vi "CV_test.vi"() -> ()   [LabVIEW 2015]
uses:
  Hardware libraries/Boonton7200/Boonton7200_IEEE-488_Bus_Mnemonics.ctl
  <vilib>/Analysis/1siggen.llb/Ramp Pattern by Delta.vi
  Hardware libraries/Boonton7200/Boonton7200.lvlib
  <vilib>/Analysis/NI_AALBase.lvlib
panel:
  in  "Zero":bool
  out "XY Graph 3":cluster{dbl[], dbl[]}(graph)
  out "XY Graph 2":cluster{dbl[], dbl[]}(graph)
  out "XY Graph":cluster{"Ramp Pattern":dbl[], dbl[]}(graph)
  out "1/C2-V":cluster{"Ramp Pattern":dbl[], dbl[]}(graph)
  out "Array":dbl[](array[numeric])
  in  "Hardware GPIB address":i32
  out "Error Out":errorcluster
  in  "Error In":errorcluster
  in  "Input parameters":T1
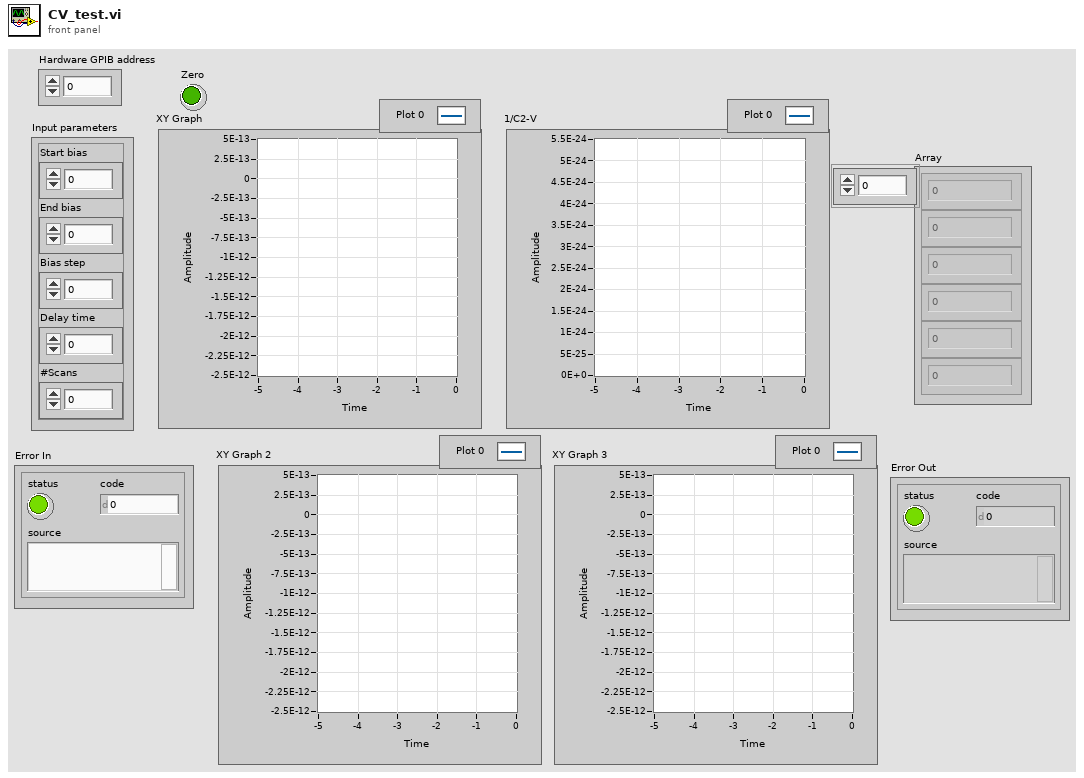
[diagram p1: front panel]
types:
  T1 = cluster{"Start bias":dbl, "End bias":dbl, "Bias step":dbl, "Delay time":u32, "#Scans":i32}
  T2 = typedef "Boonton7200_IEEE-488_Bus_Mnemonics.ctl" = string
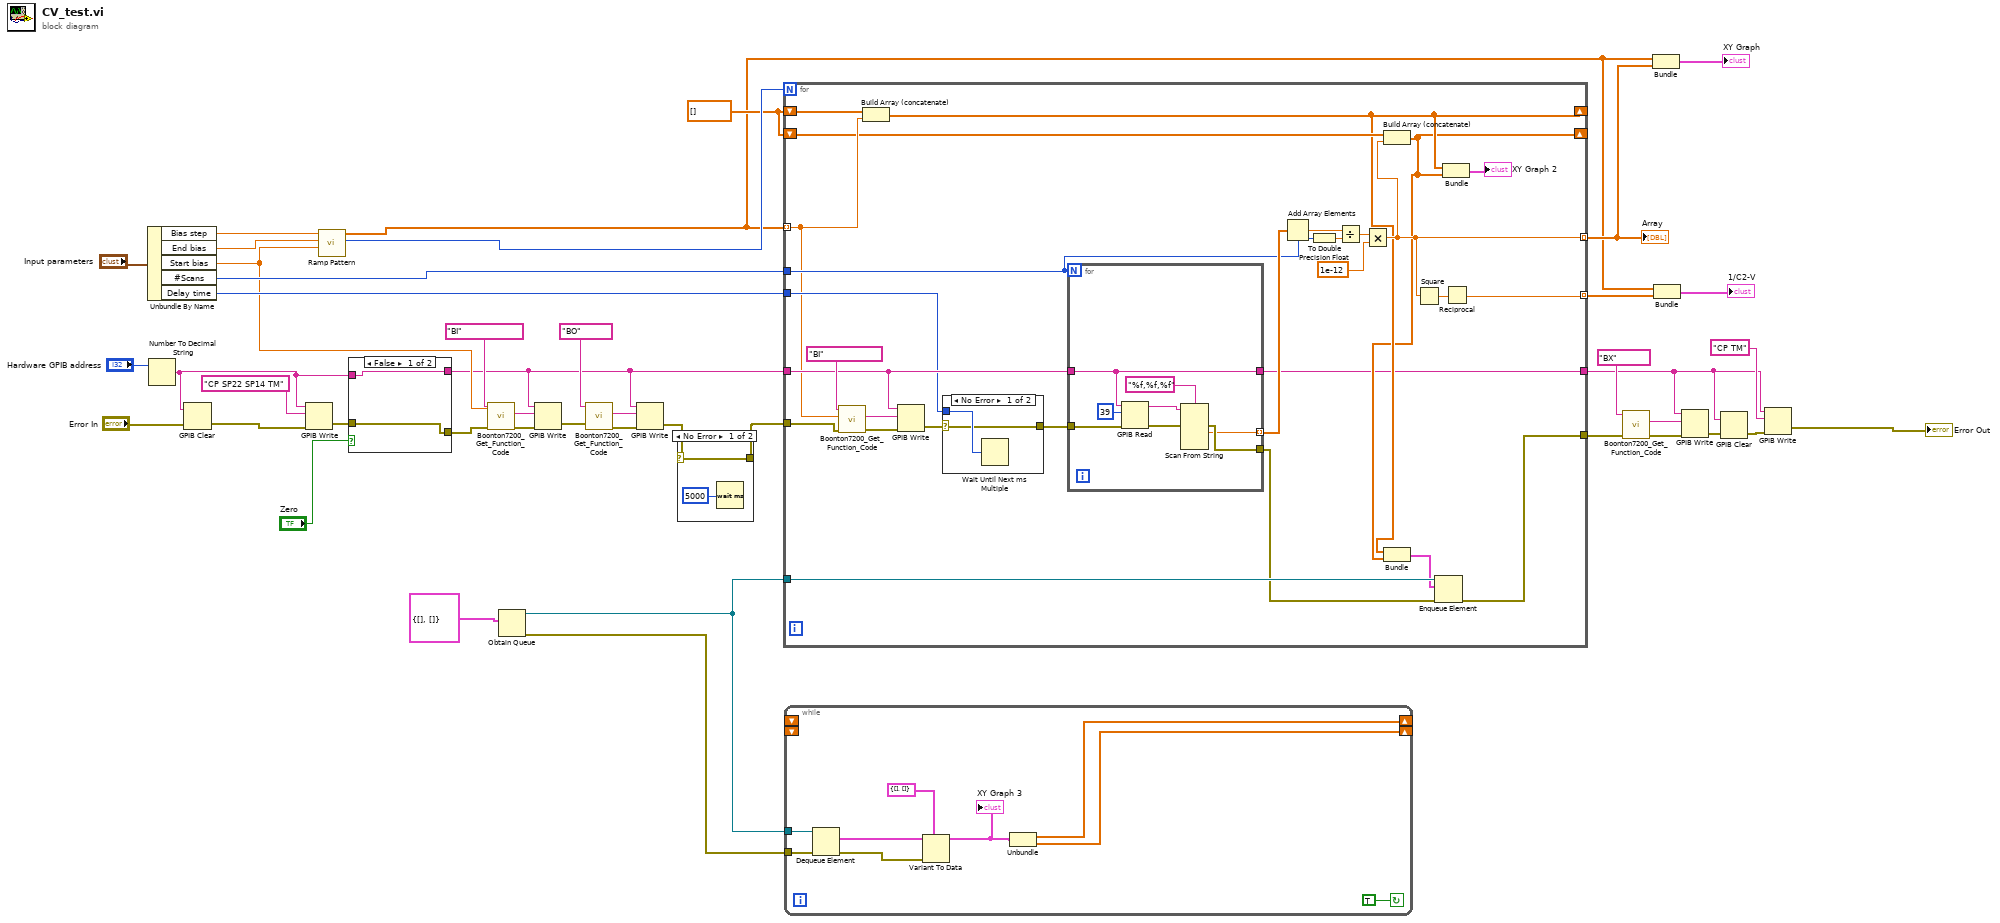
[diagram p0: block diagram]
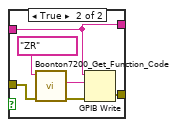
[diagram p2: hidden frame]
diagram:
  w15 = dbl[] []
  n1 = Unbundle By Name("Input parameters") -> ("Bias step"=w40:dbl, "End bias"=w39:dbl, "Start bias"=w31:dbl, "#Scans"=w37:i32, "Delay time"=w36:u32)
  n2 = Number To Decimal String(number="Hardware GPIB address") -> (decimal integer string=w3:string)  [unwired: 1 in]
  n3 = GPIB Clear(2:"Error In", 3:w3) -> (0:w34:errorcluster)  [unwired: 1 out]
  n4 = GPIB Write(0:w3, 1:"CP SP22 SP14 TM" ("data"), 3:w34) -> (6:w6:errorcluster)  [unwired: 2 in, 1 out]
  n5 = call-poly <vilib>:"Ramp Pattern.vi"("start"=w31, "end"=w39, "delta"=w40) -> ("samples"=w38:i32, "Ramp Pattern"=w12:dbl[])  [unwired: 6 in, 1 out]
  n6 = case shown="False" "Zero" {
    tunnel: w6 -> [w44 w50]
    tunnel: [w44 w48] -> w5
    tunnel: [w45 w47] -> w4
    tunnel: w3 -> [w45 w47]
    frame False {
    }
    frame True {
      n7 = call "Boonton7200_Get_Function_Code.vi"("Error In"=w50, "IEEE-488 Bus Mnemonics"=T2 "ZR") -> ("Error Out"=w49:errorcluster, "GPIB code (IEEE-488)"=w46:string)  [unwired: 8 in]
      n8 = GPIB Write(0:w47, 1:w46, 3:w49) -> (6:w48:errorcluster)  [unwired: 2 in, 1 out]
    }
  }
  n9 = call "Boonton7200_Get_Function_Code.vi"("Error In"=w5, "Data Value"=w31, "IEEE-488 Bus Mnemonics"=T2 "BI") -> ("Error Out"=w33:errorcluster, "GPIB code (IEEE-488)"=w23:string)  [unwired: 7 in]
  n10 = Obtain Queue(element data type=cluster{dbl[], dbl[]} {[], []}) -> (queue out=w14:refnum<queue>, error out=w13:errorcluster)  [unwired: 4 in, 1 out]
  n11 = GPIB Write(0:w4, 1:w23, 3:w33) -> (6:w30:errorcluster)  [unwired: 2 in, 1 out]
  n12 = call "Boonton7200_Get_Function_Code.vi"("Error In"=w30, "IEEE-488 Bus Mnemonics"=T2 "BO") -> ("Error Out"=w28:errorcluster, "GPIB code (IEEE-488)"=w22:string)  [unwired: 8 in]
  n13 = GPIB Write(0:w4, 1:w22, 3:w28) -> (6:w8:errorcluster)  [unwired: 2 in, 1 out]
  n14 = case shown="No Error" w8 {
    selector: w8 -> [w53 w54]
    tunnel: [w53 w54] -> w9
    frame No Error {
      n15 = Wait (ms)(milliseconds to wait=u32 5000) -> ()  [unwired: 1 out]
    }
    frame Error {
    }
  }
  n16 = for {
    N: w38 -> [_]
    tunnel: w12 -> [w65] mode=indexing
    tunnel: w37 -> [w75]
    tunnel: w36 -> [w71]
    tunnel: w4 -> [w79]
    tunnel: w9 -> [w78]
    tunnel: [w61] -> w27 mode=indexing
    tunnel: [w70] -> w24 mode=indexing
    shift-right: [w59] -> _
    shift-left: w15 -> [w66]
    shift-right: [w58] -> _
    shift-left: w15 -> [w64]
    tunnel: w14 -> [w62]
    tunnel: [w56] -> w10
    tunnel: [w55] -> w1
    n17 = call "Boonton7200_Get_Function_Code.vi"("Error In"=w78, "Data Value"=w65, "IEEE-488 Bus Mnemonics"=T2 "BI") -> ("Error Out"=w80:errorcluster, "GPIB code (IEEE-488)"=w74:string)  [unwired: 7 in]
    n18 = Build Array (concatenate)(w66, w65) -> (w59:dbl[])
    n19 = GPIB Write(0:w79, 1:w74, 3:w80) -> (6:w73:errorcluster)  [unwired: 2 in, 1 out]
    n20 = case shown="No Error" w73 {
      selector: w73 -> [w82 w84]
      tunnel: [w82 w84] -> w72
      tunnel: w71 -> [w83 _]
      frame No Error {
        n21 = Wait Until Next ms Multiple(millisecond multiple=w83) -> ()  [unwired: 1 out]
      }
      frame Error {
      }
    }
    n22 = for {
      N: w75 -> [_]
      tunnel: w72 -> [w92]
      tunnel: w79 -> [w85]
      tunnel: [w86] -> w77 mode=indexing
      tunnel: [w87] -> w60
      tunnel: [w85] -> w56
      n23 = GPIB Read(0:w85, 1:39 ("byte count"), 3:w92) -> (5:w90:string, 7:w88:errorcluster)  [unwired: 2 in, 1 out]
      n24 = Scan From String(format string="%f,%f,%f", input string=w90, error in=w88) -> (error out=w87:errorcluster, output 1=w86:dbl)  [unwired: 6 in, 2 out]
    }
    n25 = Add Array Elements(numeric array=w77) -> (sum=w76:dbl)
    n26 = To Double Precision Float(number=w75) -> (double precision float=w67:dbl)
    n27 = Divide(x=w76, y=w67) -> (x/y=w69:dbl)
    n28 = Multiply(x=w69, y=1e-12) -> (x*y=w61:dbl)
    n29 = Build Array (concatenate)(w64, w61) -> (w58:dbl[])
    n30 = Bundle(w59, w58) -> (w57:cluster{dbl[], dbl[]})  [unwired: 1 in]
    n31 = Square(x=w61) -> (x^2=w70:dbl)
    n32 = Enqueue Element(queue=w62, element=w57, error in (no error)=w60) -> (error out=w55:errorcluster)  [unwired: 1 in, 2 out]
    n33 = Bundle(w59, w58) -> (→"XY Graph 2":cluster{dbl[], dbl[]})  [unwired: 1 in]
    n34 = Reciprocal(x=w70) -> ()  [unwired: 1 out]
  }
  "Array" <- w27
  n35 = while {
    tunnel: w14 -> [w101]
    tunnel: w13 -> [w100]
    shift-right: [w95] -> _
    shift-left: _ -> [_]
    shift-right: [w94] -> _
    shift-left: _ -> [_]
    stop <- TRUE continue-if-true
    n36 = Dequeue Element(queue=w101, error in (no error)=w100) -> (element=w98:cluster{dbl[], dbl[]}, error out=w99:errorcluster)  [unwired: 1 in, 2 out]
    n37 = Variant To Data(error in=w99, type=cluster{dbl[], dbl[]} {[], []}, Variant=w98) -> (data=w96:cluster{dbl[], dbl[]})  [unwired: 1 out]
    "XY Graph 3" <- w96
    n38 = Unbundle(w96) -> (w94:dbl[], w95:dbl[])
  }
  n39 = call "Boonton7200_Get_Function_Code.vi"("Error In"=w1, "IEEE-488 Bus Mnemonics"=T2 "BX") -> ("Error Out"=w26:errorcluster, "GPIB code (IEEE-488)"=w21:string)  [unwired: 8 in]
  n40 = Bundle("Ramp Pattern"=w12, w27) -> (→"XY Graph":cluster{"Ramp Pattern":dbl[], dbl[]})  [unwired: 1 in]
  n41 = Bundle("Ramp Pattern"=w12, w24) -> (→"1/C2-V":cluster{"Ramp Pattern":dbl[], dbl[]})  [unwired: 1 in]
  n42 = GPIB Write(0:w10, 1:w21, 3:w26) -> (6:w18:errorcluster)  [unwired: 2 in, 1 out]
  n43 = GPIB Clear(2:w18, 3:w10) -> (0:w19:errorcluster)  [unwired: 1 out]
  n44 = GPIB Write(0:w10, 1:"CP TM" ("data"), 3:w19) -> (6:→"Error Out":errorcluster)  [unwired: 2 in, 1 out]
